vi "Actor Destroy.vi"(11 "Self Actor in":refnum<class "Self Actor.lvclass">) -> (0 "error out":errorcluster, 3 "Self Actor out":refnum<class "Self Actor.lvclass">)   [LabVIEW 2021, in "LVCAM.lvlib" / "Self Actor.lvclass"]
uses:
  Self Actor.lvclass
  Self Actor.lvclass/Self Actor.ctl
  Destroying Self Actor State/Destroying Self Actor State.lvclass
  C:/PPLs/LabVIEW-Composed-Actor-Model-LVCAM/LabVIEW-Composed-Actor-Model-LVCAM/LVCAM/LVCAM/Self Actor State/Self Actor State.lvclass
  Self Actor State/Self Actor State.lvclass
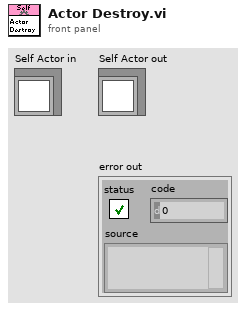
[diagram p1: front panel]
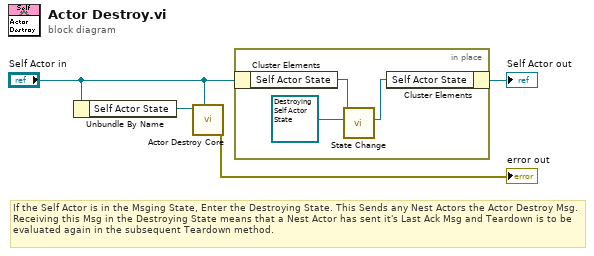
[diagram p0: block diagram]
diagram:
  # "If the Self Actor is in the Msging State, Enter the Destroying State. This Sends any Nest Actors the Actor Destroy Msg. Receiving this Msg in the Destroying State means that a Nest Actor has sent it's Last Ack Msg and Teardown is to be evaluated again in the subsequent Teardown method."
  n1 = Unbundle By Name("Self Actor in") -> ("Self Actor State"=w3:refnum<class "Self Actor State.lvclass">)
  n2 = call-dynamic "Actor Destroy Core.vi"("Self Actor in"="Self Actor in", "Self Actor State in"=w3) -> ("error out"=→"error out":errorcluster)  [unwired: 9 in]
  n3 = in-place {
    n4 = in-place-cluster #1("Self Actor in") -> ("Self Actor State"=w6:refnum<class "Self Actor State.lvclass">)
    n5 = call "State Change.vi"("Self Actor State Transition"=refnum<class "Destroying Self Actor State.lvclass"> refnum ("LVCAM.lvlib:Destroying Self Actor State.lvclass"), "Self Actor State Current"=w6) -> ("Self Actor State out"=w5:refnum<class "Destroying Self Actor State.lvclass">)  [unwired: 9 in]
    n6 = in-place-cluster #1("Self Actor State"=w5) -> (→"Self Actor out":refnum<class "Self Actor.lvclass">)
  }
